vi "Perform Action.vi"(8 "error in (no error)":errorcluster, 10 "Input":variant, 11 "Virt Voltage Generator in":refnum<class "Virt Voltage Generator.lvclass">) -> (0 "error out":errorcluster, 2 "Output":variant, 3 "Virt Voltage Generator out":refnum<class "Virt Voltage Generator.lvclass">)   [LabVIEW 2023]
uses:
  Virt Voltage Generator.lvclass
  Virt Instrument Base/Virt Instr Base.lvclass
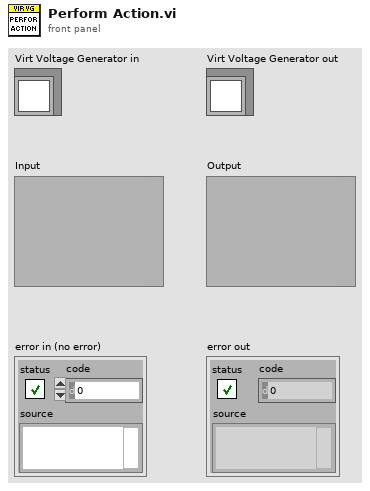
[diagram p1: front panel]
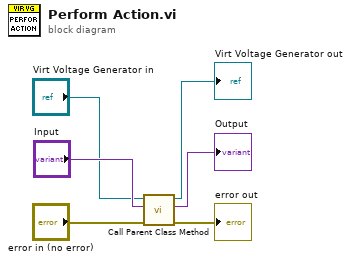
[diagram p0: block diagram]
diagram:
  n1 = call-parent "Call Parent Class Method"("error in (no error)"="error in (no error)", "Input"="Input", "Virt Instrument Base in"="Virt Voltage Generator in") -> ("error out"=→"error out":errorcluster, "Output"=→"Output":variant, "Virt Instrument Base out"=→"Virt Voltage Generator out":refnum<class "Virt Voltage Generator.lvclass">)  [unwired: 6 in]
